vi "PotentialGraph1D.vi"(8 "number":dbl, 9 "Setpoint":dbl, 10 "k":dbl, 11 "Function":string) -> (1 "potential":dbl)   [LabVIEW 2023]
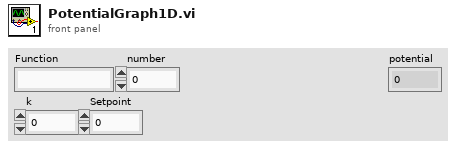
[diagram p1: front panel]
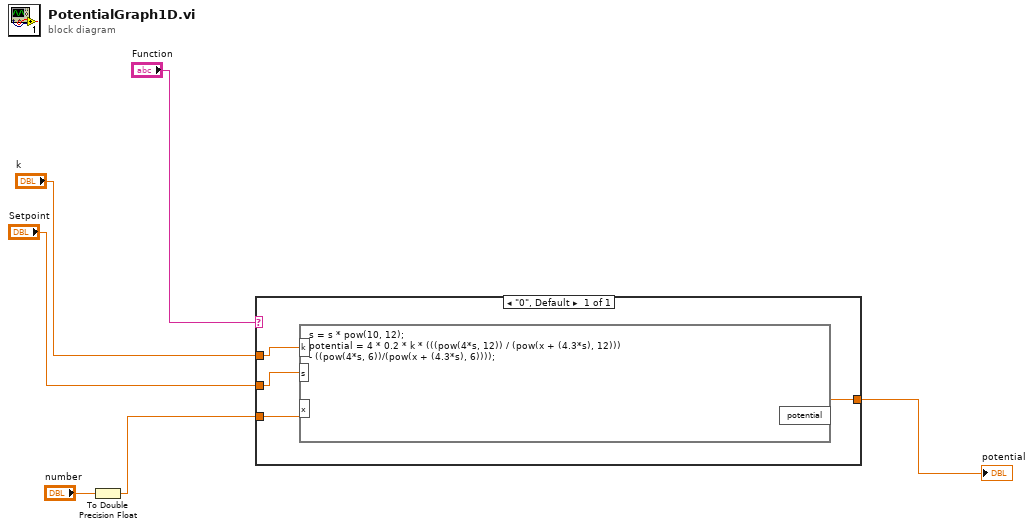
[diagram p0: block diagram]
diagram:
  n1 = To Double Precision Float(number="number") -> (double precision float=w3:dbl)
  n2 = case shown="\"0\", Default" "Function" {
    tunnel: [w9] -> w1
    tunnel: w3 -> [w10]
    tunnel: "Setpoint" -> [w7]
    tunnel: "k" -> [w8]
    frame "0", Default {
      n3 = formula code="s = s * pow(10, 12);\npotential = 4 * 0.2 * k * (((pow(4*s, 12)) / (pow(x + (4.3*s), 12))) \n- ((pow(4*s, 6))/(pow(x + (4.3*s), 6))));"("x"=w10, "s"=w7, "k"=w8) -> ("potential"=w9:dbl)
    }
  }
  "potential" <- w1
